vi "Core.vi"() -> (19 "Error Out":errorcluster)   [LabVIEW 2017]
uses:
  <vilib>/Platform/TimedLoop/XDataNode/timing_clust.ctl
  <vilib>/Platform/TimedLoop/XDataNode/nitl_modes.ctl
  <vilib>/Platform/TimedLoop/XDataNode/wakeup.ctl
  <vilib>/Platform/TimedLoop/XDataNode/XDataNode.xnode
  <vilib>/Platform/TimedLoop/XDataNode/XDNodeRunTimeDep.lvlib
panel:
  out "Output Resistance":dbl
  out "Output Resistance":dbl
  # "Core Module DIagnostics"
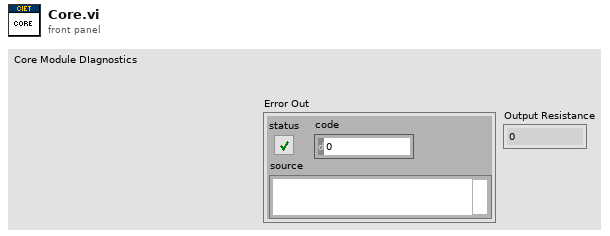
[diagram p1: front panel]
types:
  T1 = typedef "XDNodeRunTimeDep.lvlib/timing_clust.ctl" = cluster{"Expected End [f-1]":u64, "Actual End [f-1]":u64, "Finished Late? [f-1]":bool, "Expected End [i-1]":u64, "Actual End [i-1]":u64, "Finished Late? [i-1]":bool, "Expected Start [i]":u64, "Actual Start [i]":u64, "Expected Start [f]":u64, "Actual Start [f]":u64, "Source Name":string, "Structure Name":string, "Period":i64, "Deadline":i64, "Offset":i64, "Start":i64, "Priority":i32, "Timeout":i32, "Mode":T2, "Wakeup Reason":T3, "Error":errorcluster, "Source Type":string, "Secondary Source Type":string, "Global End Time":u64, "Global Start Time":u64, "Frame Duration":u64, "Iteration Duration":u64, "Assigned CPU":i32, "I/O Scan Engine Mode":u32}
  T2 = typedef "XDNodeRunTimeDep.lvlib/nitl_modes.ctl" = enum32{"No Change", "Process missed periods, maintain original phase", "Discard missed periods, maintain original phase", "Process missed periods, ignore original phase", "Discard missed periods, ignore original phase"}
  T3 = typedef "XDNodeRunTimeDep.lvlib/wakeup.ctl" = enum32{"Normal", "Aborted", "Asynchronous wakeup", "Timing source error", "Timed loop error", "Timeout"}
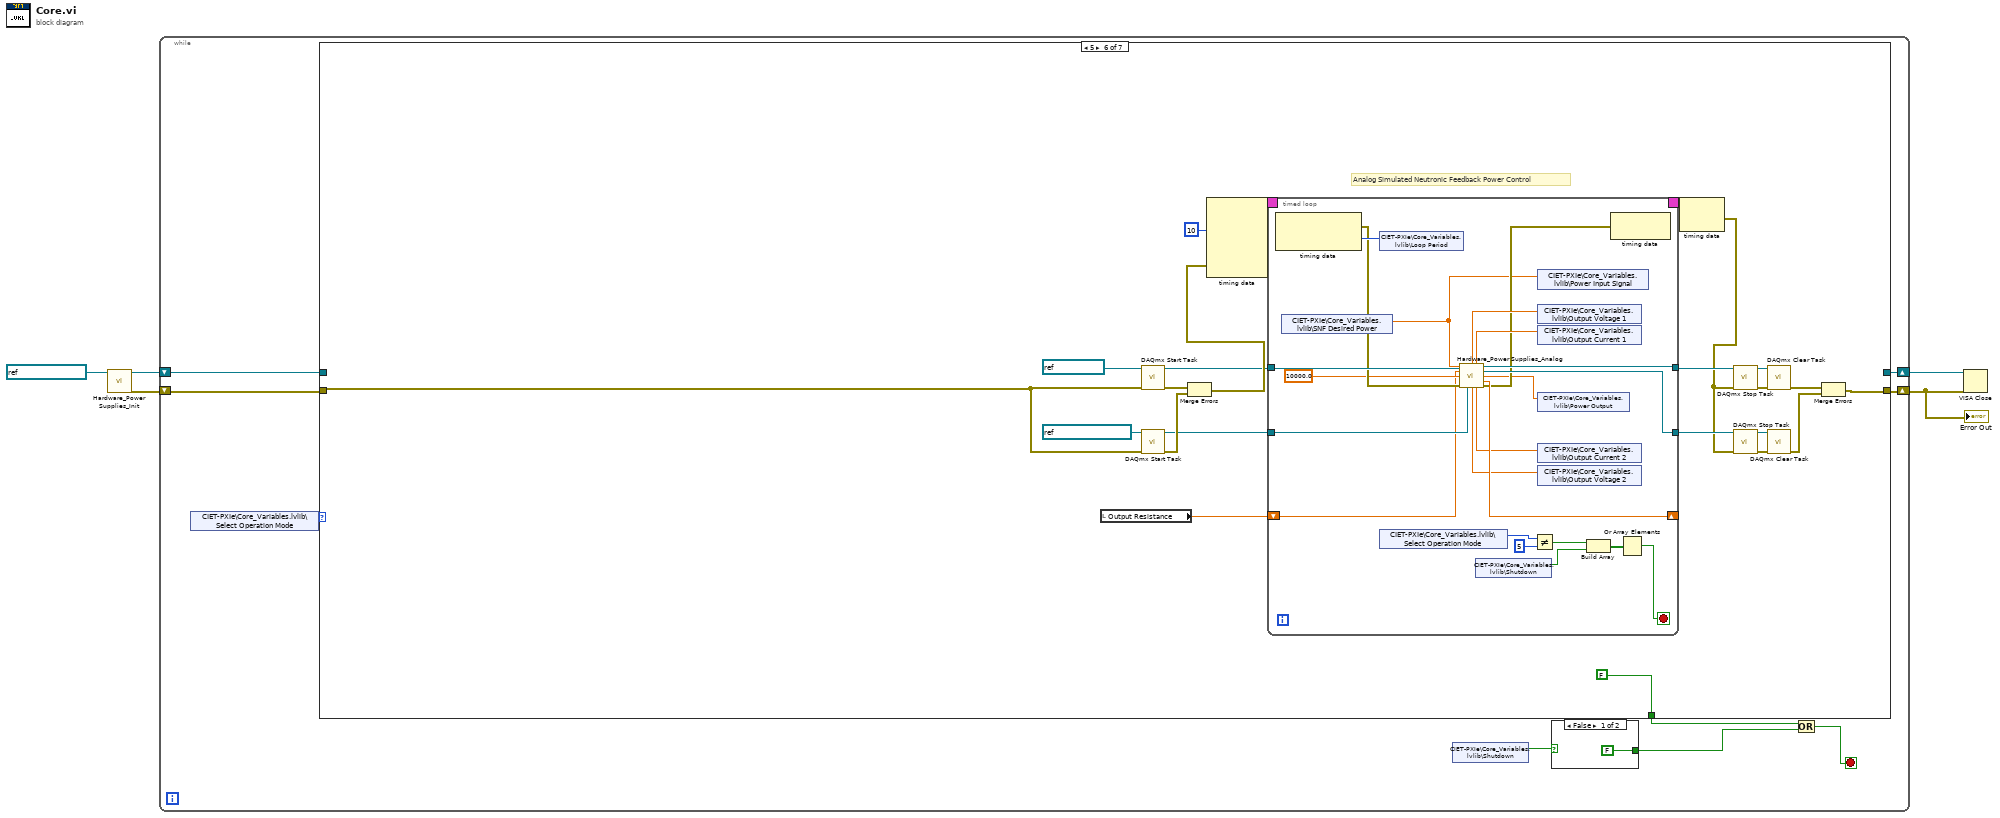
[diagram p0: block diagram]
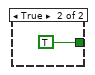
[diagram p2: hidden frame]
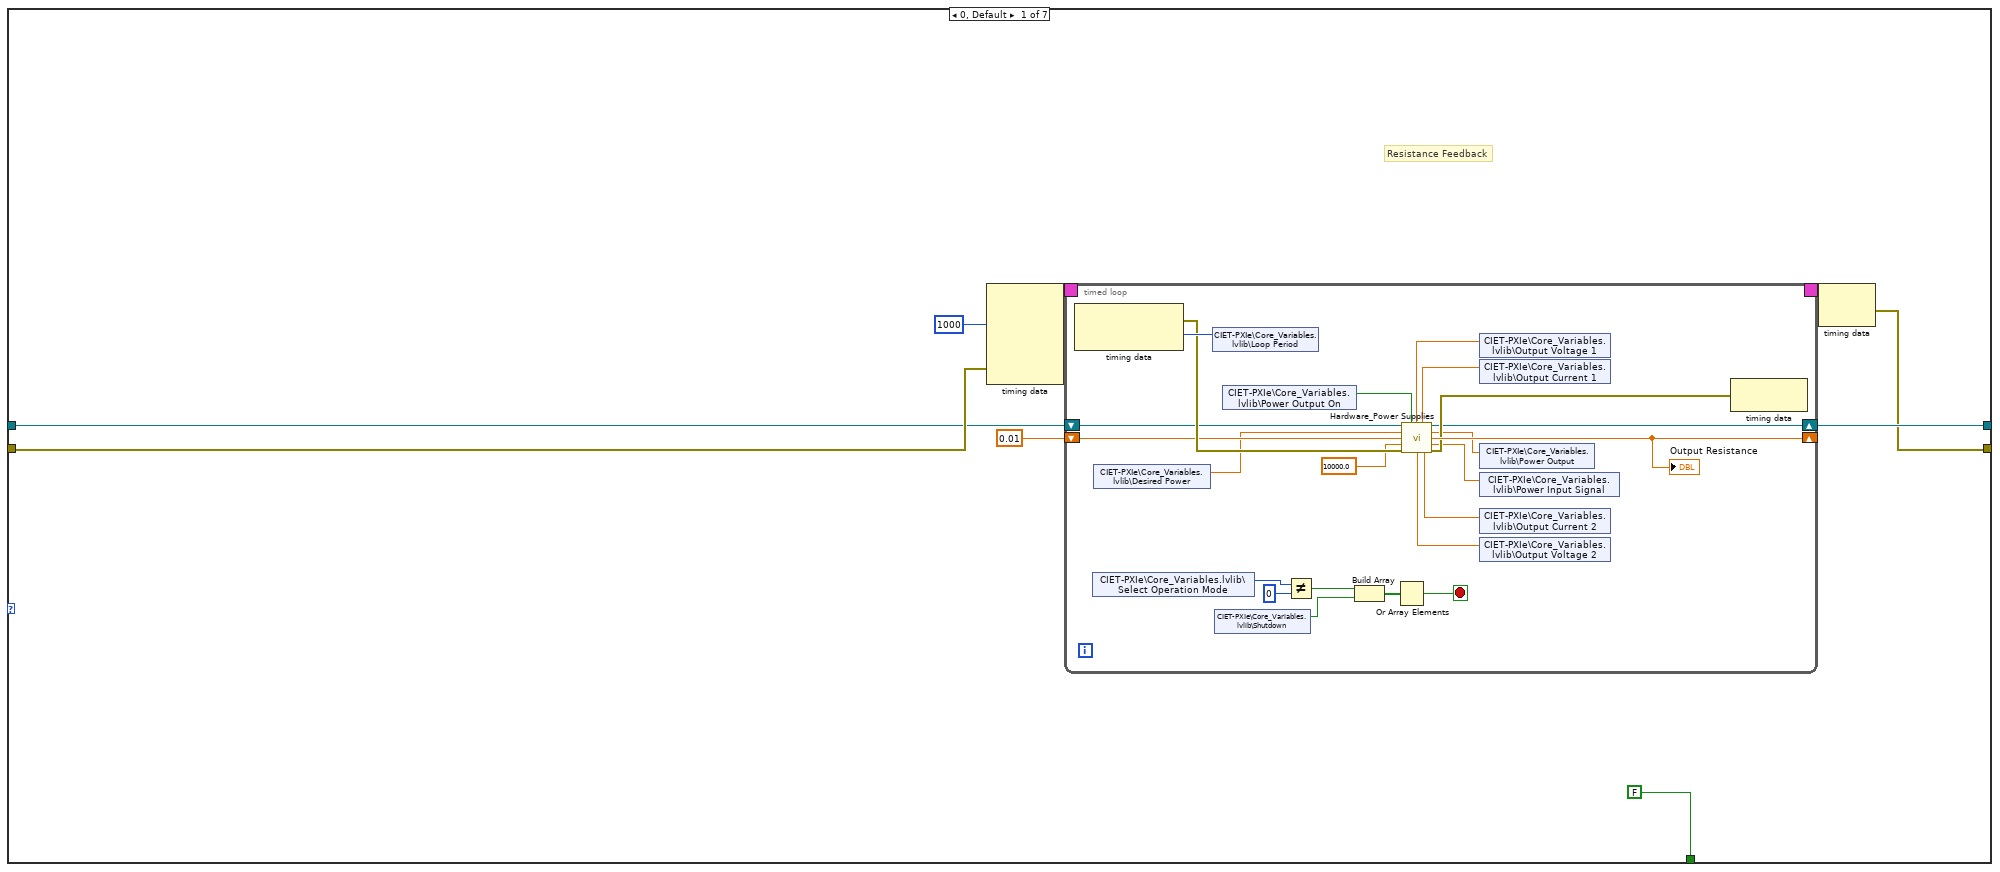
[diagram p3: hidden frame]
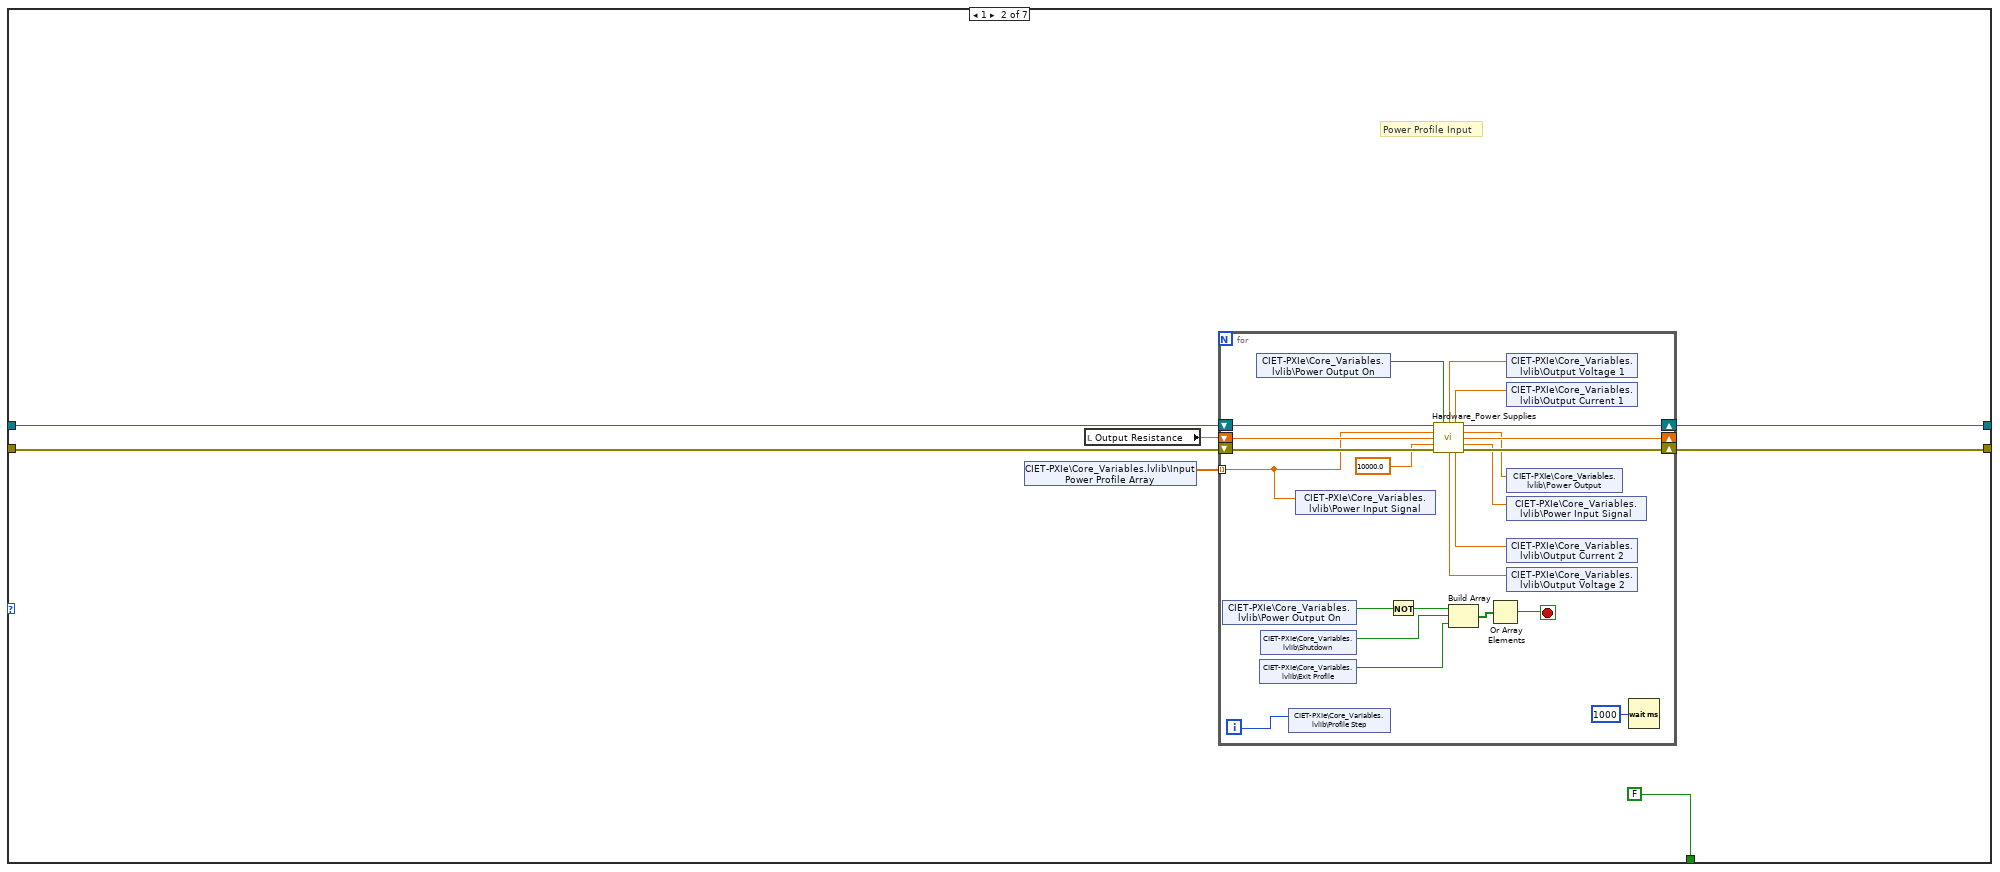
[diagram p4: hidden frame]
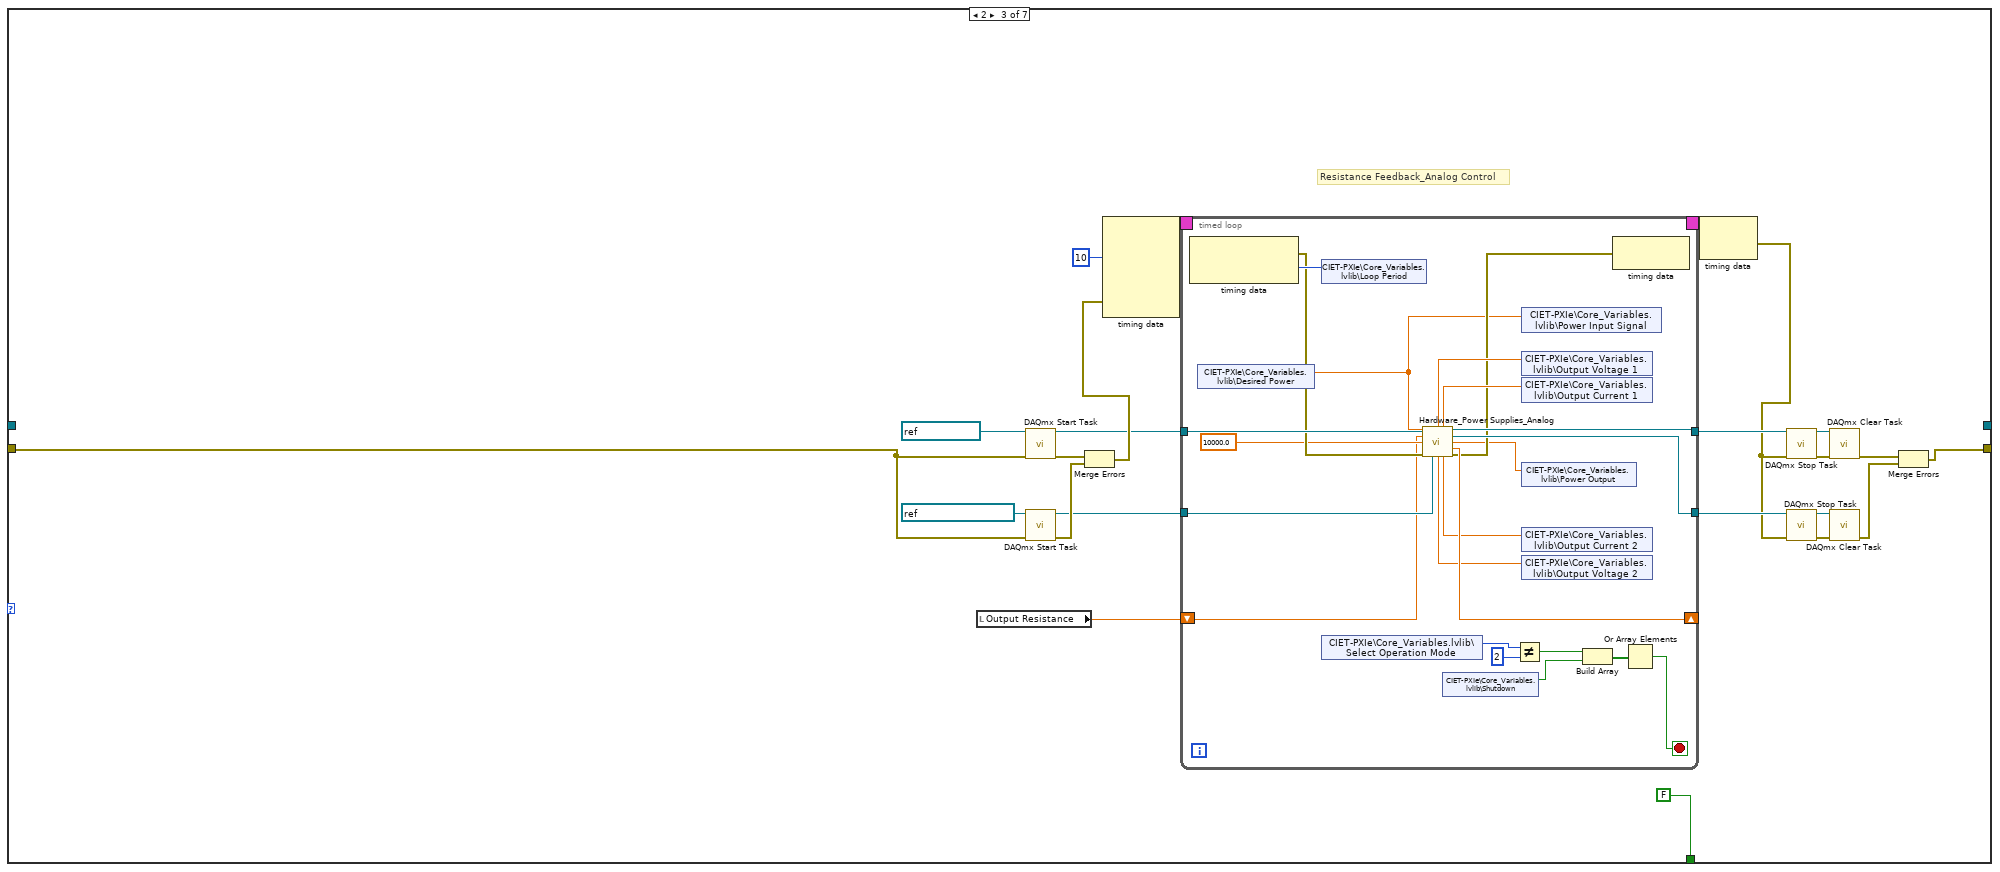
[diagram p5: hidden frame]
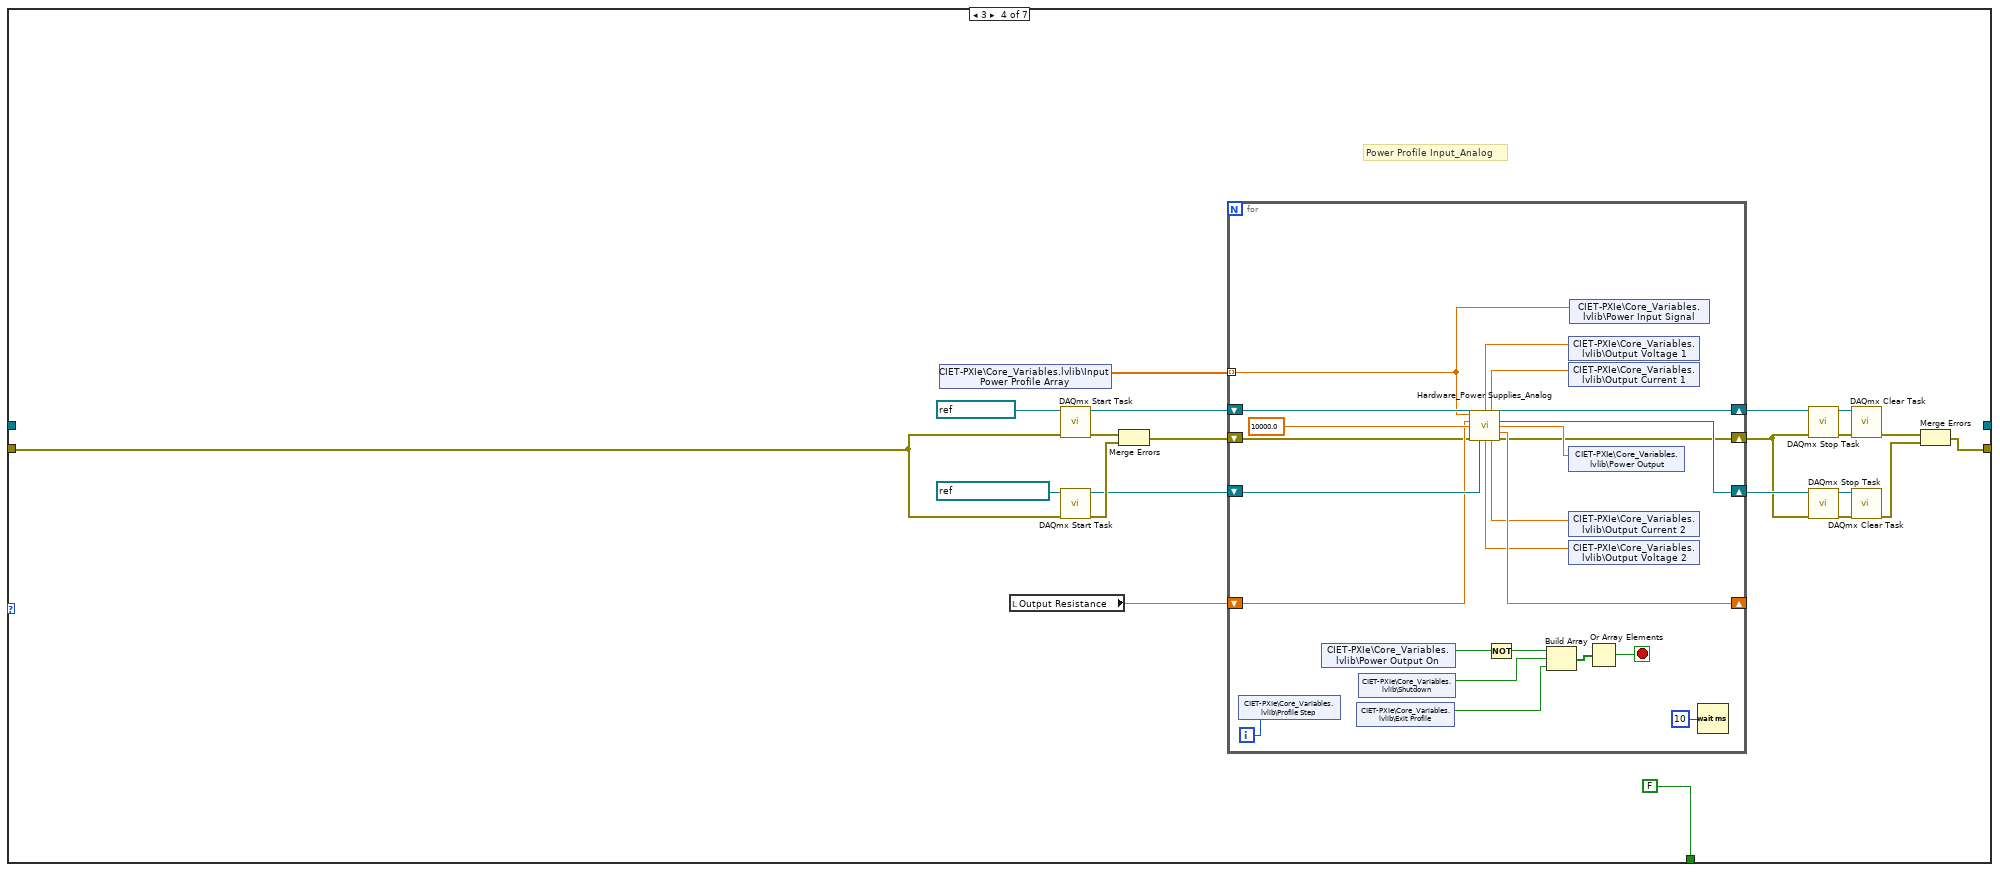
[diagram p6: hidden frame]
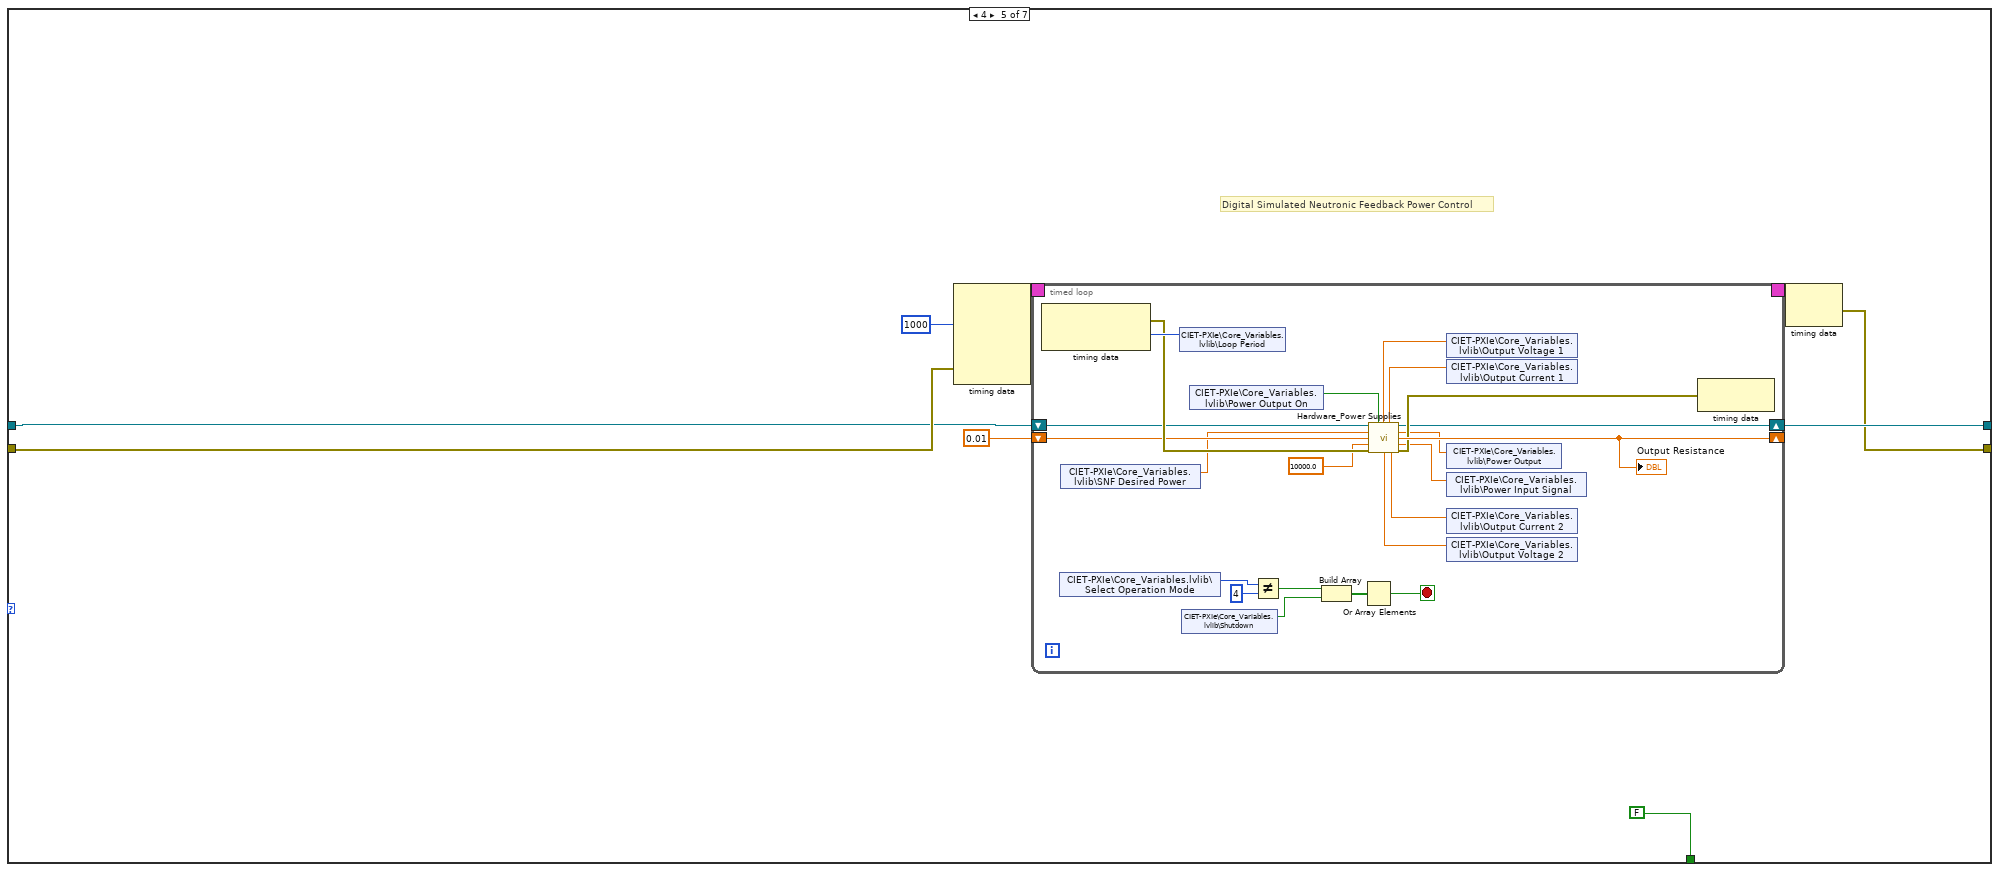
[diagram p7: hidden frame]
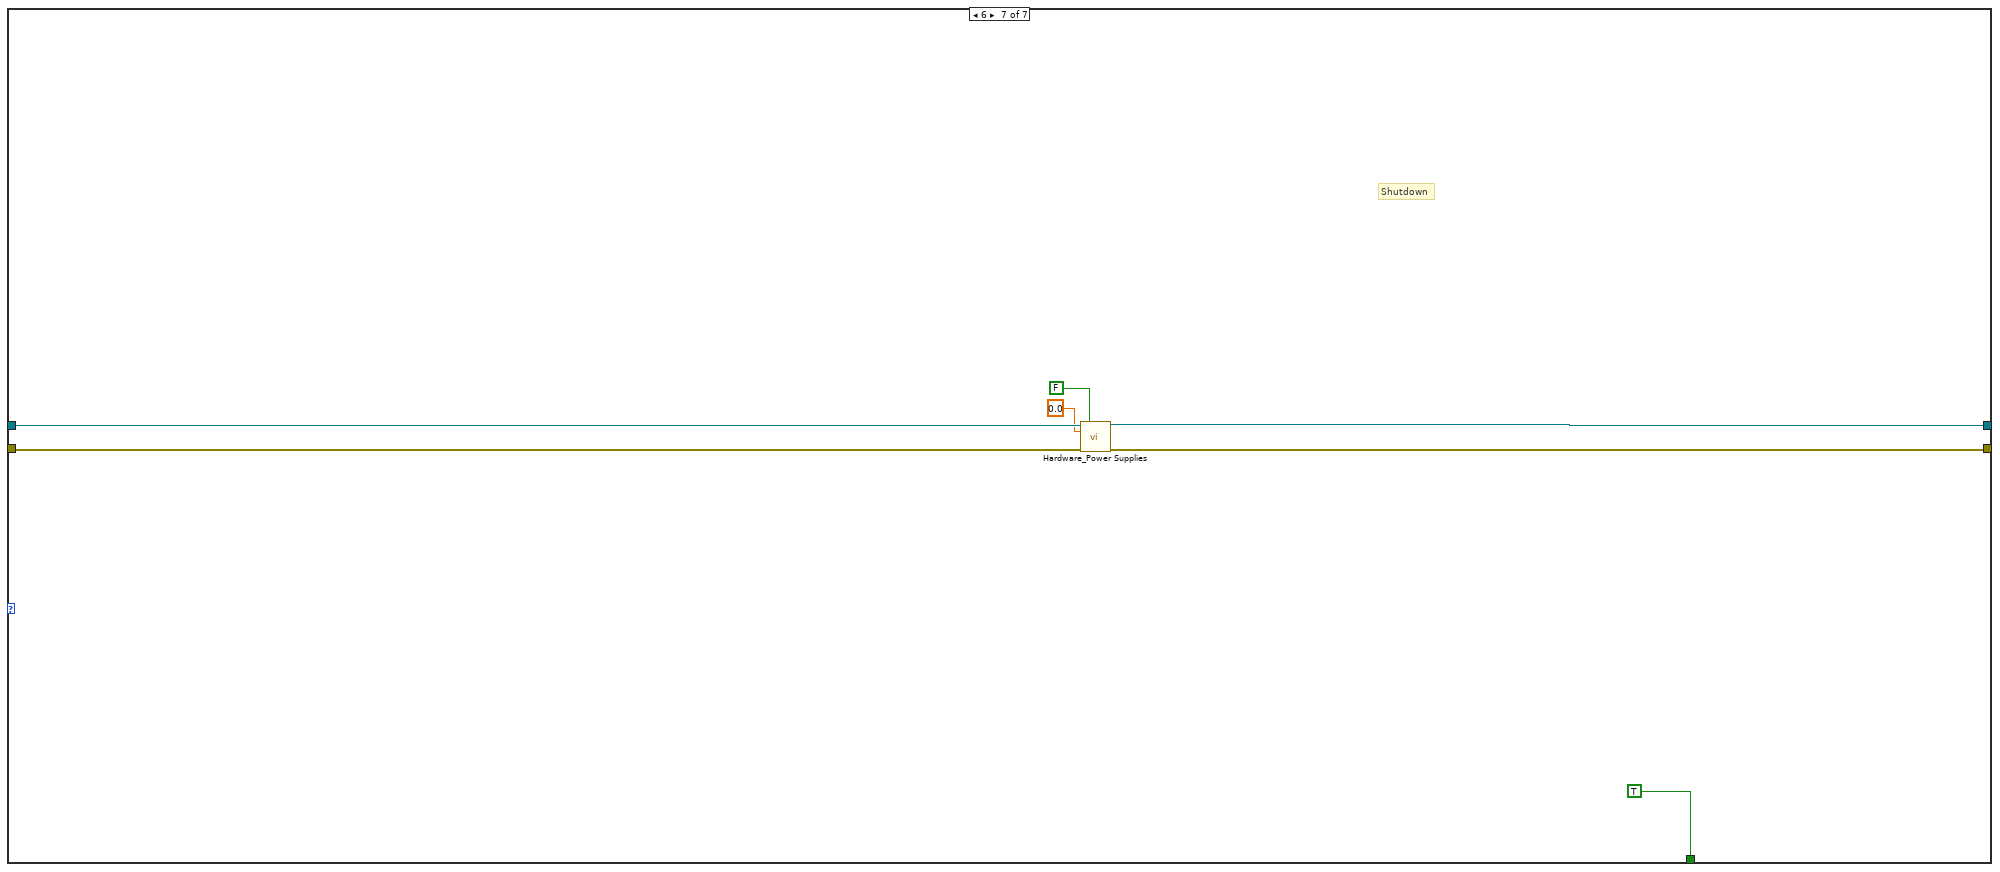
[diagram p8: hidden frame]
diagram:
  n1 = call "Hardware_Power Supplies_Init.vi"("VISA name"=refnum<visa-resource-name> "PowerSupplies") -> ("Error out"=w1:errorcluster, "VISA out"=w2:refnum<visa-resource-name>)  [unwired: 9 in]
  n2 = while {
    shift-right: [w11] -> w4
    shift-left: w1 -> [w14]
    shift-right: [w12] -> w5
    shift-left: w2 -> [w13]
    stop <- w6 stop-if-true
    n3 = shared-variable "CIET-PXIe\\Core_Variables.lvlib\\Select Operation Mode"() -> (w10:u16)  [unwired: 1 in, 1 out]
    n4 = case shown="5" w10 {
      tunnel: w14 -> [w23 w63 w97 w152 w193 w234 w296]
      tunnel: w13 -> [w22 w66 _ _ w192 _ w295]
      tunnel: [w20 w65 _ _ w195 _ w294] -> w12
      tunnel: [w19 w62 w102 w151 w194 w236 w293] -> w11
      tunnel: [FALSE ("Shutdown") FALSE ("Shutdown") FALSE ("Shutdown") FALSE ("Shutdown") FALSE ("Shutdown") FALSE ("Shutdown") TRUE ("Shutdown")] -> w8
      frame 0, Default {
        # "Resistance Feedback"
        n5 = node-c288(i64 1000 ("Period"), w23) -> (w25:T1)  [unwired: 3 in]
        n6 = timed-loop {
          timing: w25 -> [_]
          timing-out: [_] -> w24
          shift-right: [w32] -> w20
          shift-left: w22 -> [w39]
          shift-right: [w36] -> _
          shift-left: 0.01 -> [w38]
          stop <- w44 stop-if-true
          n7 = node-c288() -> (w40:errorcluster, w43:i64)  [unwired: 1 in]
          n8 = shared-variable "CIET-PXIe\\Core_Variables.lvlib\\Select Operation Mode"() -> (w42:u16)  [unwired: 1 in, 1 out]
          n9 = shared-variable "CIET-PXIe\\Core_Variables.lvlib\\Desired Power"() -> (w26:dbl)  [unwired: 1 in, 1 out]
          n10 = shared-variable "CIET-PXIe\\Core_Variables.lvlib\\Loop Period"(w43) -> ()  [unwired: 1 in, 1 out]
          n11 = shared-variable "CIET-PXIe\\Core_Variables.lvlib\\Shutdown"() -> (w41:bool)  [unwired: 1 in, 1 out]
          n12 = shared-variable "CIET-PXIe\\Core_Variables.lvlib\\Power Output On"() -> (w31:bool)  [unwired: 1 in, 1 out]
          n13 = Not Equal?(x=w42, y=u16 0) -> (x != y?=w46:bool)
          n14 = Build Array(w46, w41) -> (w45:bool[])
          n15 = Or Array Elements(Boolean array=w45) -> (logical OR=w44:bool)
          n16 = call "Hardware_Power Supplies.vi"("Input VISA"=w39, "Power Output ON"=w31, "Desired Power"=w26, "Input Resistance"=w38, "Maximum Power Limit"=10000.0, "Input Error"=w40) -> ("Output Voltage 1"=w30:dbl, "Output Current 1"=w29:dbl, "Output VISA"=w32:refnum<visa-resource-name>, "Output Power"=w33:dbl, "Output Resistance"=w36:dbl, "Input Power"=w34:dbl, "Output Voltage 2"=w27:dbl, "Output Current 2"=w28:dbl, "Output Error"=w35:errorcluster)  [unwired: 1 in]
          "Output Resistance" <- w36
          n17 = shared-variable "CIET-PXIe\\Core_Variables.lvlib\\Output Voltage 1"(w30) -> ()  [unwired: 1 in, 1 out]
          n18 = shared-variable "CIET-PXIe\\Core_Variables.lvlib\\Output Current 1"(w29) -> ()  [unwired: 1 in, 1 out]
          n19 = shared-variable "CIET-PXIe\\Core_Variables.lvlib\\Power Output"(w33) -> ()  [unwired: 1 in, 1 out]
          n20 = shared-variable "CIET-PXIe\\Core_Variables.lvlib\\Power Input Signal"(w34) -> ()  [unwired: 1 in, 1 out]
          n21 = shared-variable "CIET-PXIe\\Core_Variables.lvlib\\Output Current 2"(w28) -> ()  [unwired: 1 in, 1 out]
          n22 = shared-variable "CIET-PXIe\\Core_Variables.lvlib\\Output Voltage 2"(w27) -> ()  [unwired: 1 in, 1 out]
          n23 = node-c288(w35) -> ()  [unwired: 1 out]
        }
        n24 = node-c288(w24) -> (w19:errorcluster)
      }
      frame 1 {
        # "Power Profile Input"
        n25 = shared-variable "CIET-PXIe\\Core_Variables.lvlib\\Input Power Profile Array"() -> (w60:dbl[])  [unwired: 1 in, 1 out]
        n26 = local read "Output Resistance"() -> (w64:dbl)
        n27 = for {
          shift-right: [w81] -> w65
          shift-left: w66 -> [w82]
          shift-right: [w80] -> w62
          shift-left: w63 -> [w79]
          tunnel: w60 -> [w67] mode=indexing
          shift-right: [w73] -> _
          shift-left: w64 -> [w72]
          i -> [w83]
          stop <- w87 stop-if-true
          n28 = shared-variable "CIET-PXIe\\Core_Variables.lvlib\\Power Output On"() -> (w85:bool)  [unwired: 1 in, 1 out]
          n29 = shared-variable "CIET-PXIe\\Core_Variables.lvlib\\Power Output On"() -> (w78:bool)  [unwired: 1 in, 1 out]
          n30 = shared-variable "CIET-PXIe\\Core_Variables.lvlib\\Exit Profile"() -> (w68:bool)  [unwired: 1 in, 1 out]
          n31 = shared-variable "CIET-PXIe\\Core_Variables.lvlib\\Shutdown"() -> (w84:bool)  [unwired: 1 in, 1 out]
          n32 = shared-variable "CIET-PXIe\\Core_Variables.lvlib\\Profile Step"(w83) -> ()  [unwired: 1 in, 1 out]
          n33 = shared-variable "CIET-PXIe\\Core_Variables.lvlib\\Power Input Signal"(w67) -> ()  [unwired: 1 in, 1 out]
          n34 = Not(x=w85) -> (.not. x?=w86:bool)
          n35 = call "Hardware_Power Supplies.vi"("Input VISA"=w82, "Power Output ON"=w78, "Desired Power"=w67, "Input Resistance"=w72, "Maximum Power Limit"=10000.0, "Input Error"=w79) -> ("Output Voltage 1"=w77:dbl, "Output Current 1"=w76:dbl, "Output VISA"=w81:refnum<visa-resource-name>, "Output Power"=w70:dbl, "Output Resistance"=w73:dbl, "Input Power"=w69:dbl, "Output Voltage 2"=w75:dbl, "Output Current 2"=w74:dbl, "Output Error"=w80:errorcluster)  [unwired: 1 in]
          n36 = Build Array(w86, w84, w68) -> (w89:bool[])
          n37 = Or Array Elements(Boolean array=w89) -> (logical OR=w87:bool)
          n38 = shared-variable "CIET-PXIe\\Core_Variables.lvlib\\Output Voltage 1"(w77) -> ()  [unwired: 1 in, 1 out]
          n39 = shared-variable "CIET-PXIe\\Core_Variables.lvlib\\Output Current 1"(w76) -> ()  [unwired: 1 in, 1 out]
          n40 = shared-variable "CIET-PXIe\\Core_Variables.lvlib\\Power Output"(w70) -> ()  [unwired: 1 in, 1 out]
          n41 = shared-variable "CIET-PXIe\\Core_Variables.lvlib\\Power Input Signal"(w69) -> ()  [unwired: 1 in, 1 out]
          n42 = shared-variable "CIET-PXIe\\Core_Variables.lvlib\\Output Current 2"(w74) -> ()  [unwired: 1 in, 1 out]
          n43 = shared-variable "CIET-PXIe\\Core_Variables.lvlib\\Output Voltage 2"(w75) -> ()  [unwired: 1 in, 1 out]
          n44 = Wait (ms)(milliseconds to wait=u32 1000) -> ()  [unwired: 1 out]
        }
      }
      frame 2 {
        # "Resistance Feedback_Analog Control"
        n45 = local read "Output Resistance"() -> (w94:dbl)
        n46 = call <vilib>:"DAQmx Start Task.vi"("task/channels in"=refnum<k21> "PowerOut", "error in"=w97) -> ("task out"=w96:refnum<k21>, "error out"=w112:errorcluster)  [unwired: 12 in]
        n47 = call <vilib>:"DAQmx Start Task.vi"("task/channels in"=refnum<k21> "PowerMonitor_V", "error in"=w97) -> ("task out"=w95:refnum<k21>, "error out"=w111:errorcluster)  [unwired: 12 in]
        n48 = Merge Errors(w112, w111) -> (w98:errorcluster)
        n49 = node-c288(i64 10 ("Period"), w98) -> (w101:T1)  [unwired: 3 in]
        n50 = timed-loop {
          timing: w101 -> [_]
          timing-out: [_] -> w100
          shift-right: [w128] -> _
          shift-left: w94 -> [w129]
          tunnel: w96 -> [w133]
          tunnel: [w127] -> w93
          tunnel: w95 -> [w132]
          tunnel: [w126] -> w92
          stop <- w114 stop-if-true
          n51 = node-c288() -> (w131:errorcluster, w134:i64)  [unwired: 1 in]
          n52 = shared-variable "CIET-PXIe\\Core_Variables.lvlib\\Desired Power"() -> (w113:dbl)  [unwired: 1 in, 1 out]
          n53 = shared-variable "CIET-PXIe\\Core_Variables.lvlib\\Loop Period"(w134) -> ()  [unwired: 1 in, 1 out]
          n54 = shared-variable "CIET-PXIe\\Core_Variables.lvlib\\Select Operation Mode"() -> (w116:u16)  [unwired: 1 in, 1 out]
          n55 = call "Hardware_Power Supplies_Analog.vi"("Desired Power"=w113, "Task In_1"=w133, "Input Resistance"=w129, "Maximum Power Limit"=10000.0, "Error In"=w131, "Task In_2"=w132) -> ("Output Voltage 1"=w125:dbl, "Output Current 1"=w124:dbl, "Task Out_1"=w127:refnum<k21>, "Task Out_2"=w126:refnum<k21>, "Output Power"=w120:dbl, "Output Resistance"=w128:dbl, "Output Voltage 2"=w123:dbl, "Output Current 2"=w122:dbl, "Error Out"=w121:errorcluster)  [unwired: 1 in]
          n56 = shared-variable "CIET-PXIe\\Core_Variables.lvlib\\Shutdown"() -> (w115:bool)  [unwired: 1 in, 1 out]
          n57 = Not Equal?(x=w116, y=u16 2) -> (x != y?=w118:bool)
          n58 = shared-variable "CIET-PXIe\\Core_Variables.lvlib\\Power Input Signal"(w113) -> ()  [unwired: 1 in, 1 out]
          n59 = shared-variable "CIET-PXIe\\Core_Variables.lvlib\\Output Voltage 1"(w125) -> ()  [unwired: 1 in, 1 out]
          n60 = shared-variable "CIET-PXIe\\Core_Variables.lvlib\\Output Current 1"(w124) -> ()  [unwired: 1 in, 1 out]
          n61 = shared-variable "CIET-PXIe\\Core_Variables.lvlib\\Power Output"(w120) -> ()  [unwired: 1 in, 1 out]
          n62 = shared-variable "CIET-PXIe\\Core_Variables.lvlib\\Output Current 2"(w122) -> ()  [unwired: 1 in, 1 out]
          n63 = shared-variable "CIET-PXIe\\Core_Variables.lvlib\\Output Voltage 2"(w123) -> ()  [unwired: 1 in, 1 out]
          n64 = Build Array(w118, w115) -> (w117:bool[])
          n65 = node-c288(w121) -> ()  [unwired: 1 out]
          n66 = Or Array Elements(Boolean array=w117) -> (logical OR=w114:bool)
        }
        n67 = node-c288(w100) -> (w90:errorcluster)
        n68 = call <vilib>:"DAQmx Stop Task.vi"("task/channels in"=w93, "error in"=w90) -> ("task out"=w108:refnum<k21>, "error out"=w107:errorcluster)  [unwired: 12 in]
        n69 = call <vilib>:"DAQmx Stop Task.vi"("task/channels in"=w92, "error in"=w90) -> ("task out"=w106:refnum<k21>, "error out"=w105:errorcluster)  [unwired: 12 in]
        n70 = call <vilib>:"DAQmx Clear Task.vi"("task in"=w108, "error in"=w107) -> ("error out"=w104:errorcluster)  [unwired: 13 in]
        n71 = call <vilib>:"DAQmx Clear Task.vi"("task in"=w106, "error in"=w105) -> ("error out"=w103:errorcluster)  [unwired: 13 in]
        n72 = Merge Errors(w104, w103) -> (w102:errorcluster)
      }
      frame 3 {
        # "Power Profile Input_Analog"
        n73 = shared-variable "CIET-PXIe\\Core_Variables.lvlib\\Input Power Profile Array"() -> (w148:dbl[])  [unwired: 1 in, 1 out]
        n74 = local read "Output Resistance"() -> (w155:dbl)
        n75 = call <vilib>:"DAQmx Start Task.vi"("task/channels in"=refnum<k21> "PowerOut", "error in"=w152) -> ("task out"=w157:refnum<k21>, "error out"=w167:errorcluster)  [unwired: 12 in]
        n76 = call <vilib>:"DAQmx Start Task.vi"("task/channels in"=refnum<k21> "PowerMonitor_V", "error in"=w152) -> ("task out"=w156:refnum<k21>, "error out"=w166:errorcluster)  [unwired: 12 in]
        n77 = Merge Errors(w167, w166) -> (w150:errorcluster)
        n78 = for {
          shift-right: [w186] -> _
          shift-left: w155 -> [w187]
          shift-right: [w185] -> w154
          shift-left: w157 -> [w190]
          shift-right: [w184] -> w153
          shift-left: w156 -> [w189]
          shift-right: [w177] -> w149
          shift-left: w150 -> [w178]
          tunnel: w148 -> [w168] mode=indexing
          i -> [w172]
          stop <- w171 stop-if-true
          n79 = shared-variable "CIET-PXIe\\Core_Variables.lvlib\\Profile Step"(w172) -> ()  [unwired: 1 in, 1 out]
          n80 = shared-variable "CIET-PXIe\\Core_Variables.lvlib\\Power Output On"() -> (w174:bool)  [unwired: 1 in, 1 out]
          n81 = shared-variable "CIET-PXIe\\Core_Variables.lvlib\\Exit Profile"() -> (w169:bool)  [unwired: 1 in, 1 out]
          n82 = shared-variable "CIET-PXIe\\Core_Variables.lvlib\\Shutdown"() -> (w173:bool)  [unwired: 1 in, 1 out]
          n83 = call "Hardware_Power Supplies_Analog.vi"("Desired Power"=w168, "Task In_1"=w190, "Input Resistance"=w187, "Maximum Power Limit"=10000.0, "Error In"=w178, "Task In_2"=w189) -> ("Output Voltage 1"=w183:dbl, "Output Current 1"=w182:dbl, "Task Out_1"=w185:refnum<k21>, "Task Out_2"=w184:refnum<k21>, "Output Power"=w179:dbl, "Output Resistance"=w186:dbl, "Output Voltage 2"=w181:dbl, "Output Current 2"=w180:dbl, "Error Out"=w177:errorcluster)  [unwired: 1 in]
          n84 = Not(x=w174) -> (.not. x?=w175:bool)
          n85 = Build Array(w175, w173, w169) -> (w176:bool[])
          n86 = shared-variable "CIET-PXIe\\Core_Variables.lvlib\\Output Voltage 1"(w183) -> ()  [unwired: 1 in, 1 out]
          n87 = shared-variable "CIET-PXIe\\Core_Variables.lvlib\\Output Current 1"(w182) -> ()  [unwired: 1 in, 1 out]
          n88 = shared-variable "CIET-PXIe\\Core_Variables.lvlib\\Power Output"(w179) -> ()  [unwired: 1 in, 1 out]
          n89 = shared-variable "CIET-PXIe\\Core_Variables.lvlib\\Output Current 2"(w180) -> ()  [unwired: 1 in, 1 out]
          n90 = shared-variable "CIET-PXIe\\Core_Variables.lvlib\\Output Voltage 2"(w181) -> ()  [unwired: 1 in, 1 out]
          n91 = shared-variable "CIET-PXIe\\Core_Variables.lvlib\\Power Input Signal"(w168) -> ()  [unwired: 1 in, 1 out]
          n92 = Or Array Elements(Boolean array=w176) -> (logical OR=w171:bool)
          n93 = Wait (ms)(milliseconds to wait=u32 10) -> ()  [unwired: 1 out]
        }
        n94 = call <vilib>:"DAQmx Stop Task.vi"("task/channels in"=w154, "error in"=w149) -> ("task out"=w163:refnum<k21>, "error out"=w162:errorcluster)  [unwired: 12 in]
        n95 = call <vilib>:"DAQmx Stop Task.vi"("task/channels in"=w153, "error in"=w149) -> ("task out"=w161:refnum<k21>, "error out"=w160:errorcluster)  [unwired: 12 in]
        n96 = call <vilib>:"DAQmx Clear Task.vi"("task in"=w163, "error in"=w162) -> ("error out"=w159:errorcluster)  [unwired: 13 in]
        n97 = call <vilib>:"DAQmx Clear Task.vi"("task in"=w161, "error in"=w160) -> ("error out"=w158:errorcluster)  [unwired: 13 in]
        n98 = Merge Errors(w159, w158) -> (w151:errorcluster)
      }
      frame 4 {
        # "Digital Simulated Neutronic Feedback Power Control"
        n99 = node-c288(i64 1000 ("Period"), w193) -> (w199:T1)  [unwired: 3 in]
        n100 = timed-loop {
          timing: w199 -> [_]
          timing-out: [_] -> w198
          shift-right: [w206] -> w195
          shift-left: w192 -> [w213]
          shift-right: [w210] -> _
          shift-left: 0.01 -> [w212]
          stop <- w218 stop-if-true
          n101 = node-c288() -> (w214:errorcluster, w217:i64)  [unwired: 1 in]
          n102 = shared-variable "CIET-PXIe\\Core_Variables.lvlib\\Select Operation Mode"() -> (w216:u16)  [unwired: 1 in, 1 out]
          n103 = shared-variable "CIET-PXIe\\Core_Variables.lvlib\\SNF Desired Power"() -> (w200:dbl)  [unwired: 1 in, 1 out]
          n104 = shared-variable "CIET-PXIe\\Core_Variables.lvlib\\Loop Period"(w217) -> ()  [unwired: 1 in, 1 out]
          n105 = shared-variable "CIET-PXIe\\Core_Variables.lvlib\\Shutdown"() -> (w215:bool)  [unwired: 1 in, 1 out]
          n106 = shared-variable "CIET-PXIe\\Core_Variables.lvlib\\Power Output On"() -> (w205:bool)  [unwired: 1 in, 1 out]
          n107 = Not Equal?(x=w216, y=u16 4) -> (x != y?=w220:bool)
          n108 = Build Array(w220, w215) -> (w219:bool[])
          n109 = Or Array Elements(Boolean array=w219) -> (logical OR=w218:bool)
          n110 = call "Hardware_Power Supplies.vi"("Input VISA"=w213, "Power Output ON"=w205, "Desired Power"=w200, "Input Resistance"=w212, "Maximum Power Limit"=10000.0, "Input Error"=w214) -> ("Output Voltage 1"=w204:dbl, "Output Current 1"=w203:dbl, "Output VISA"=w206:refnum<visa-resource-name>, "Output Power"=w207:dbl, "Output Resistance"=w210:dbl, "Input Power"=w208:dbl, "Output Voltage 2"=w201:dbl, "Output Current 2"=w202:dbl, "Output Error"=w209:errorcluster)  [unwired: 1 in]
          "Output Resistance" <- w210
          n111 = shared-variable "CIET-PXIe\\Core_Variables.lvlib\\Output Voltage 1"(w204) -> ()  [unwired: 1 in, 1 out]
          n112 = shared-variable "CIET-PXIe\\Core_Variables.lvlib\\Output Current 1"(w203) -> ()  [unwired: 1 in, 1 out]
          n113 = shared-variable "CIET-PXIe\\Core_Variables.lvlib\\Power Output"(w207) -> ()  [unwired: 1 in, 1 out]
          n114 = shared-variable "CIET-PXIe\\Core_Variables.lvlib\\Power Input Signal"(w208) -> ()  [unwired: 1 in, 1 out]
          n115 = shared-variable "CIET-PXIe\\Core_Variables.lvlib\\Output Current 2"(w202) -> ()  [unwired: 1 in, 1 out]
          n116 = shared-variable "CIET-PXIe\\Core_Variables.lvlib\\Output Voltage 2"(w201) -> ()  [unwired: 1 in, 1 out]
          n117 = node-c288(w209) -> ()  [unwired: 1 out]
        }
        n118 = node-c288(w198) -> (w194:errorcluster)
      }
      frame 5 {
        # "Analog Simulated Neutronic Feedback Power Control"
        n119 = local read "Output Resistance"() -> (w240:dbl)
        n120 = call <vilib>:"DAQmx Start Task.vi"("task/channels in"=refnum<k21> "PowerOut", "error in"=w234) -> ("task out"=w242:refnum<k21>, "error out"=w254:errorcluster)  [unwired: 12 in]
        n121 = call <vilib>:"DAQmx Start Task.vi"("task/channels in"=refnum<k21> "PowerMonitor_V", "error in"=w234) -> ("task out"=w241:refnum<k21>, "error out"=w253:errorcluster)  [unwired: 12 in]
        n122 = Merge Errors(w254, w253) -> (w243:errorcluster)
        n123 = node-c288(i64 10 ("Period"), w243) -> (w256:T1)  [unwired: 3 in]
        n124 = timed-loop {
          timing: w256 -> [_]
          timing-out: [_] -> w255
          shift-right: [w272] -> _
          shift-left: w240 -> [w273]
          tunnel: w242 -> [w277]
          tunnel: [w271] -> w239
          tunnel: w241 -> [w276]
          tunnel: [w270] -> w238
          stop <- w258 stop-if-true
          n125 = node-c288() -> (w275:errorcluster, w278:i64)  [unwired: 1 in]
          n126 = shared-variable "CIET-PXIe\\Core_Variables.lvlib\\SNF Desired Power"() -> (w257:dbl)  [unwired: 1 in, 1 out]
          n127 = shared-variable "CIET-PXIe\\Core_Variables.lvlib\\Loop Period"(w278) -> ()  [unwired: 1 in, 1 out]
          n128 = shared-variable "CIET-PXIe\\Core_Variables.lvlib\\Select Operation Mode"() -> (w260:u16)  [unwired: 1 in, 1 out]
          n129 = call "Hardware_Power Supplies_Analog.vi"("Desired Power"=w257, "Task In_1"=w277, "Input Resistance"=w273, "Maximum Power Limit"=10000.0, "Error In"=w275, "Task In_2"=w276) -> ("Output Voltage 1"=w269:dbl, "Output Current 1"=w268:dbl, "Task Out_1"=w271:refnum<k21>, "Task Out_2"=w270:refnum<k21>, "Output Power"=w264:dbl, "Output Resistance"=w272:dbl, "Output Voltage 2"=w267:dbl, "Output Current 2"=w266:dbl, "Error Out"=w265:errorcluster)  [unwired: 1 in]
          n130 = shared-variable "CIET-PXIe\\Core_Variables.lvlib\\Shutdown"() -> (w259:bool)  [unwired: 1 in, 1 out]
          n131 = Not Equal?(x=w260, y=u16 5) -> (x != y?=w262:bool)
          n132 = shared-variable "CIET-PXIe\\Core_Variables.lvlib\\Power Input Signal"(w257) -> ()  [unwired: 1 in, 1 out]
          n133 = shared-variable "CIET-PXIe\\Core_Variables.lvlib\\Output Voltage 1"(w269) -> ()  [unwired: 1 in, 1 out]
          n134 = shared-variable "CIET-PXIe\\Core_Variables.lvlib\\Output Current 1"(w268) -> ()  [unwired: 1 in, 1 out]
          n135 = shared-variable "CIET-PXIe\\Core_Variables.lvlib\\Power Output"(w264) -> ()  [unwired: 1 in, 1 out]
          n136 = shared-variable "CIET-PXIe\\Core_Variables.lvlib\\Output Current 2"(w266) -> ()  [unwired: 1 in, 1 out]
          n137 = shared-variable "CIET-PXIe\\Core_Variables.lvlib\\Output Voltage 2"(w267) -> ()  [unwired: 1 in, 1 out]
          n138 = Build Array(w262, w259) -> (w261:bool[])
          n139 = node-c288(w265) -> ()  [unwired: 1 out]
          n140 = Or Array Elements(Boolean array=w261) -> (logical OR=w258:bool)
        }
        n141 = node-c288(w255) -> (w237:errorcluster)
        n142 = call <vilib>:"DAQmx Stop Task.vi"("task/channels in"=w239, "error in"=w237) -> ("task out"=w250:refnum<k21>, "error out"=w249:errorcluster)  [unwired: 12 in]
        n143 = call <vilib>:"DAQmx Stop Task.vi"("task/channels in"=w238, "error in"=w237) -> ("task out"=w248:refnum<k21>, "error out"=w247:errorcluster)  [unwired: 12 in]
        n144 = call <vilib>:"DAQmx Clear Task.vi"("task in"=w250, "error in"=w249) -> ("error out"=w246:errorcluster)  [unwired: 13 in]
        n145 = call <vilib>:"DAQmx Clear Task.vi"("task in"=w248, "error in"=w247) -> ("error out"=w245:errorcluster)  [unwired: 13 in]
        n146 = Merge Errors(w246, w245) -> (w236:errorcluster)
      }
      frame 6 {
        # "Shutdown"
        n147 = call "Hardware_Power Supplies.vi"("Input VISA"=w295, "Power Output ON"=FALSE, "Desired Power"=0.0, "Input Error"=w296) -> ("Output VISA"=w294:refnum<visa-resource-name>, "Output Error"=w293:errorcluster)  [unwired: 3 in, 7 out]
      }
    }
    n148 = shared-variable "CIET-PXIe\\Core_Variables.lvlib\\Shutdown"() -> (w9:bool)  [unwired: 1 in, 1 out]
    n149 = case shown="False" w9 {
      tunnel: [FALSE ("Shutdown") TRUE ("Shutdown")] -> w7
      frame False {
      }
      frame True {
      }
    }
    n150 = Or(x=w8, y=w7) -> (x .or. y?=w6:bool)
  }
  "Error Out" <- w4
  n151 = VISA Close(VISA resource name=w5, error in (no error)=w4) -> ()  [unwired: 1 out]
